vi "Setpoint Profile Simulator.vi"() -> ()   [LabVIEW 2023]
doc: "This VI demonstrates how to specify a profile of setpoints and have the PID controller track this profile."
uses:
  <vilib>/addons/control/pid/pid.llb/PID (DBL).vi
  <vilib>/addons/control/pid/NI_PID_pid.lvlib
panel:
  out "SP:":dbl(slide)=60.7843137254902 min=0.0 max=0.0 scale=0.0..100.0
  out "MV:":dbl(slide)=18.78965245852964 scale=-100.0..100.0
  out "PV:":dbl(slide)=60.754431603254424 scale=0.0..100.0
  in  "Reinitialize Profile":bool
  out "Profile Elapsed Time (s)":dbl=15.000000000000078 format="%.3f"
  in  "Setpoint Profile":cluster{"time (s)":dbl, "setpoint":dbl}[](array[cluster])=[{"time (s)"=0.0, "setpoint"=0.0}, {"time (s)"=3.0, "setpoint"=40.0}, {"time (s)"=3.0, "setpoint"=80.0}, {"time (s)"=6.0, "setpoint"=80.0}, {"time (s)"=6.5, "setpoint"=85.0}, {"time (s)"=7.0, "setpoint"=80.0}, {"time (s)"=7.5, "setpoint"=85.0}, {"time (s)"=8.0, "setpoint"=80.0}, {"time (s)"=8.5, "setpoint"=85.0}, {"time (s)"=9.0, "setpoint"=80.0}, {"time (s)"=11.0, "setpoint"=80.0}, {"time (s)"=15.0, "setpoint"=0.0}] {"setpoint" format="%.2f"; "time (s)" format="%.3f"}
  in  "PID gains":T1={"proportional gain (Kc)"=10.0, "integral time (Ti, min)"=0.01, "derivative time (Td, min)"=0.001} {"derivative time (Td, min)" format="%.3f"; "integral time (Ti, min)" format="%.3f"; "proportional gain (Kc)" format="%.3f"}
  in  "Stop":bool
  out "PV Setpoint Output":cluster{"initial PV":dbl, "setpoint":dbl}(graph)={"initial PV"=0.18693112703744846, "setpoint"=0.0}
  # "Overview: This VI demonstrates how to specify a profile of setpoints and have the PID controller track this profile.\nInstructions:\n1. Run the VI.\n2. Verify the setpoint profile being generate and the controller tracking its value.\n3. Press the Reinitialize Profile to see the profile start again.\n4. Click Stop to stop the VI."
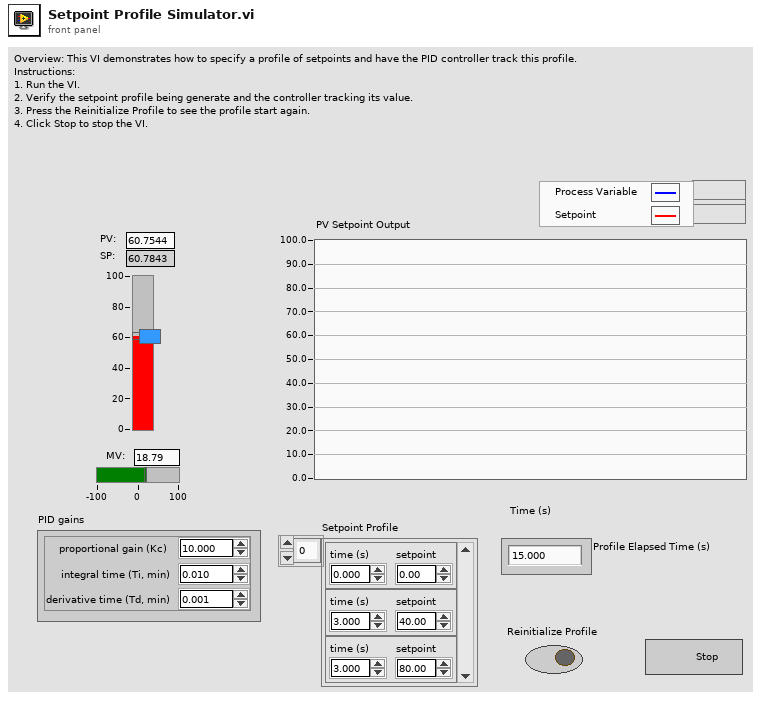
[diagram p1: front panel]
types:
  T1 = cluster{"proportional gain (Kc)":dbl, "integral time (Ti, min)":dbl, "derivative time (Td, min)":dbl}
  T2 = cluster{"static gain":dbl, "lag (min)":dbl, "dead cycles":dbl, "load %":dbl, "deadband":dbl, "noise level %":dbl, "initial PV":dbl, "initial PV 2":dbl}
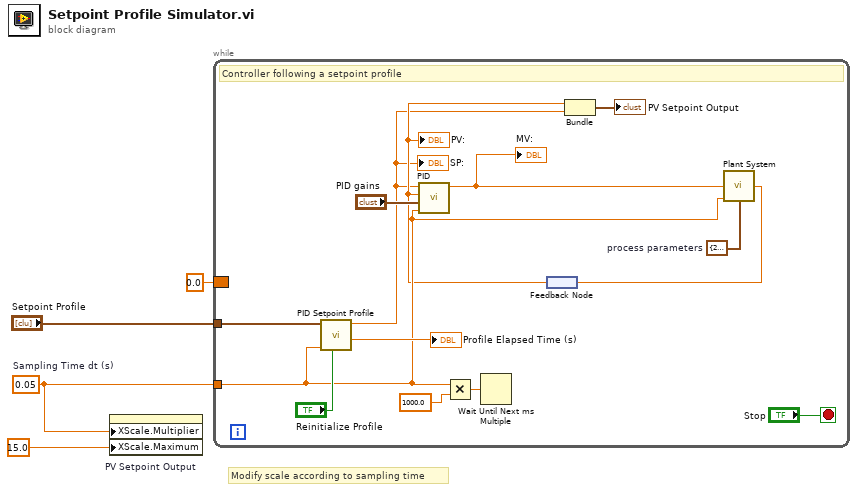
[diagram p0: block diagram]
diagram:
  w3 = 0.05  # Sampling Time dt (s)
  # "Modify scale according to sampling time"
  n1 = property on="PV Setpoint Output" class="WFChart (strict)"("XScale.Multiplier"=w3, "XScale.Maximum"=15.0 ("X Scale.Range:Maximum")) -> ()  [unwired: 2 in, 2 out]
  n2 = while {
    tunnel: "Setpoint Profile" -> [w14]
    tunnel: w3 -> [w10]
    border: 0.0 ("Plant Output") -> [_]
    stop <- "Stop" stop-if-true
    w11 = T2 {"static gain"=2.5, "lag (min)"=4.0, "dead cycles"=0.1, "load %"=40.0, "deadband"=2.0, "noise level %"=0.25, "initial PV"=0.0, "initial PV 2"=0.0}  # process parameters
    # "Controller following a setpoint profile"
    n3 = call <vilib>:"PID Setpoint Profile.vi"("reinitialize? (F)"="Reinitialize Profile", "dt (s)"=w10, "setpoint profile"=w14) -> ("elapsed time (s)"=→"Profile Elapsed Time (s)":dbl, "setpoint"=w5:dbl)  [unwired: 3 in, 2 out]
    "SP:" <- w5
    n4 = Multiply(x=w10, y=1000.0) -> (x*y=w8:dbl)
    n5 = Wait Until Next ms Multiple(millisecond multiple=w8) -> ()  [unwired: 1 out]
    n6 = feedback #1() -> (w7:dbl)
    "PV:" <- w7
    n7 = call-poly <vilib>:"PID.vi"("dt (s)"=w10, "PID gains"="PID gains", "process variable"=w7, "setpoint"=w5) -> ("output"=w6:dbl)  [unwired: 6 in, 1 out]
    "MV:" <- w6
    n8 = Bundle("Plant Output"=w7, "setpoint"=w5) -> (→"PV Setpoint Output":cluster{"Plant Output":dbl, "setpoint":dbl})  [unwired: 1 in]
    n9 = call "Plant System.vi"("Plant Input"=w6, "dt (s)"=w10, "process parameters"=w11) -> ("Plant Output"=w16:dbl)  [unwired: 12 in]
    n10 = feedback-in #1(w16) -> ()
  }
